vi "Poll.vi"(8 "error in (no error)":errorcluster, 10 "Switchable Device in":refnum<class "Switchable Device.lvclass">, 11 "Button in":refnum<class "Button.lvclass">) -> (0 "error out":errorcluster, 2 "Switchable Device out":refnum<class "Switchable Device.lvclass">, 3 "Button out":refnum<class "Button.lvclass">)   [LabVIEW 2018, in "Button.lvclass"]
uses:
  Button.lvclass
  Switchable Device/Switchable Device.lvclass
  Button.lvclass/Button.ctl
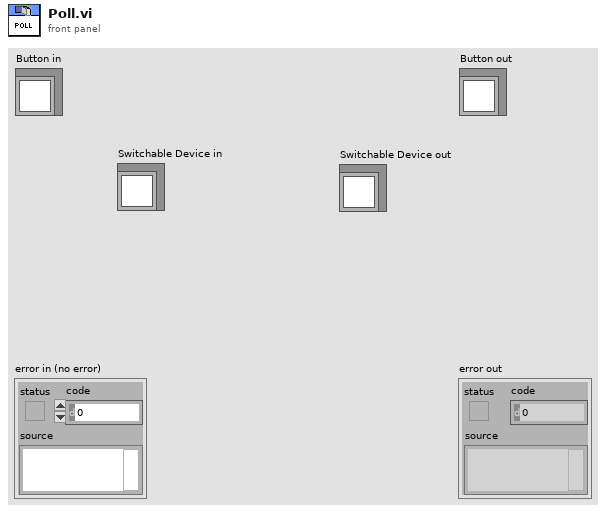
[diagram p1: front panel]
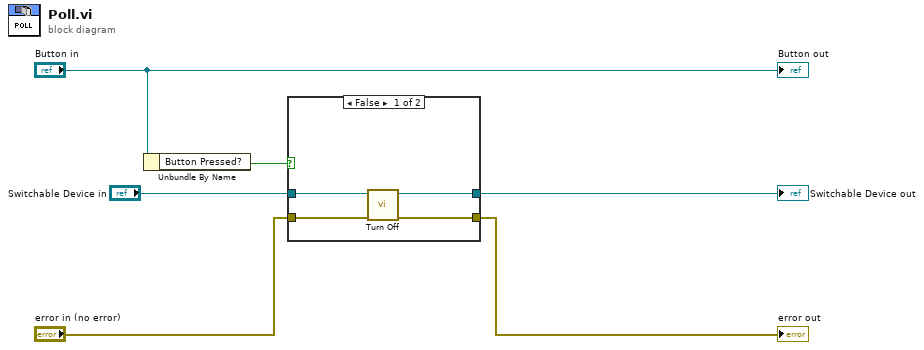
[diagram p0: block diagram]
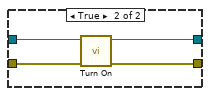
[diagram p2: hidden frame]
diagram:
  n1 = Unbundle By Name("Button in") -> ("Button Pressed?"=w5:bool)
  n2 = case shown="False" w5 {
    tunnel: "Switchable Device in" -> [w10 w13]
    tunnel: "error in (no error)" -> [w9 w14]
    tunnel: [w8 w12] -> w2
    tunnel: [w7 w11] -> w1
    frame False {
      n3 = call-dynamic "Turn Off.vi"("error in (no error)"=w9, "Switchable Device in"=w10) -> ("error out"=w8:errorcluster, "Switchable Device out"=w7:refnum<class "Switchable Device.lvclass">)  [unwired: 8 in]
    }
    frame True {
      n4 = call-dynamic "Turn On.vi"("error in (no error)"=w14, "Switchable Device in"=w13) -> ("error out"=w12:errorcluster, "Switchable Device out"=w11:refnum<class "Switchable Device.lvclass">)  [unwired: 8 in]
    }
  }
  "error out" <- w2
  "Switchable Device out" <- w1
  "Button out" <- "Button in"
